vi "Drive Controller.vi"(8 "error in":errorcluster) -> ()   [LabVIEW 2015]
doc: "This VI executes continuously carrying out the current operation and responding to updates or new operation requests. It will often contain the timing or control code that is difficult to place directly in TeleOp. This VI generally opens all sensors and motors and isolates the rest of the robot code from knowing implementation details of how the operations are carried out."
uses:
  <vilib>/Rock Robotics/WPI/CAN/TalonSRX/WPI_CANTalonSRX_GlobalStatus.ctl
  Drive Setpoints.ctl
  Drive Operations.ctl
  <vilib>/Rock Robotics/WPI/CAN/TalonSRX/WPI_CANTalonSRX_APIControlMode.ctl
  <vilib>/Rock Robotics/WPI/SafetyOutput/WPI_SafetyOutputConfigMenu.ctl
  <vilib>/Rock Robotics/WPI/MotorControl/WPI_MotorControlOpenCANTalonSRX.vi
panel:
  out "Talon SRX Status":T1
  out "Setpoints":T2(graph)
  out "Current\nCmd":string
  # "Tip: It may be helpful to observe inputs and sensor values.\nYou may also want to display tuning or debugging controls."
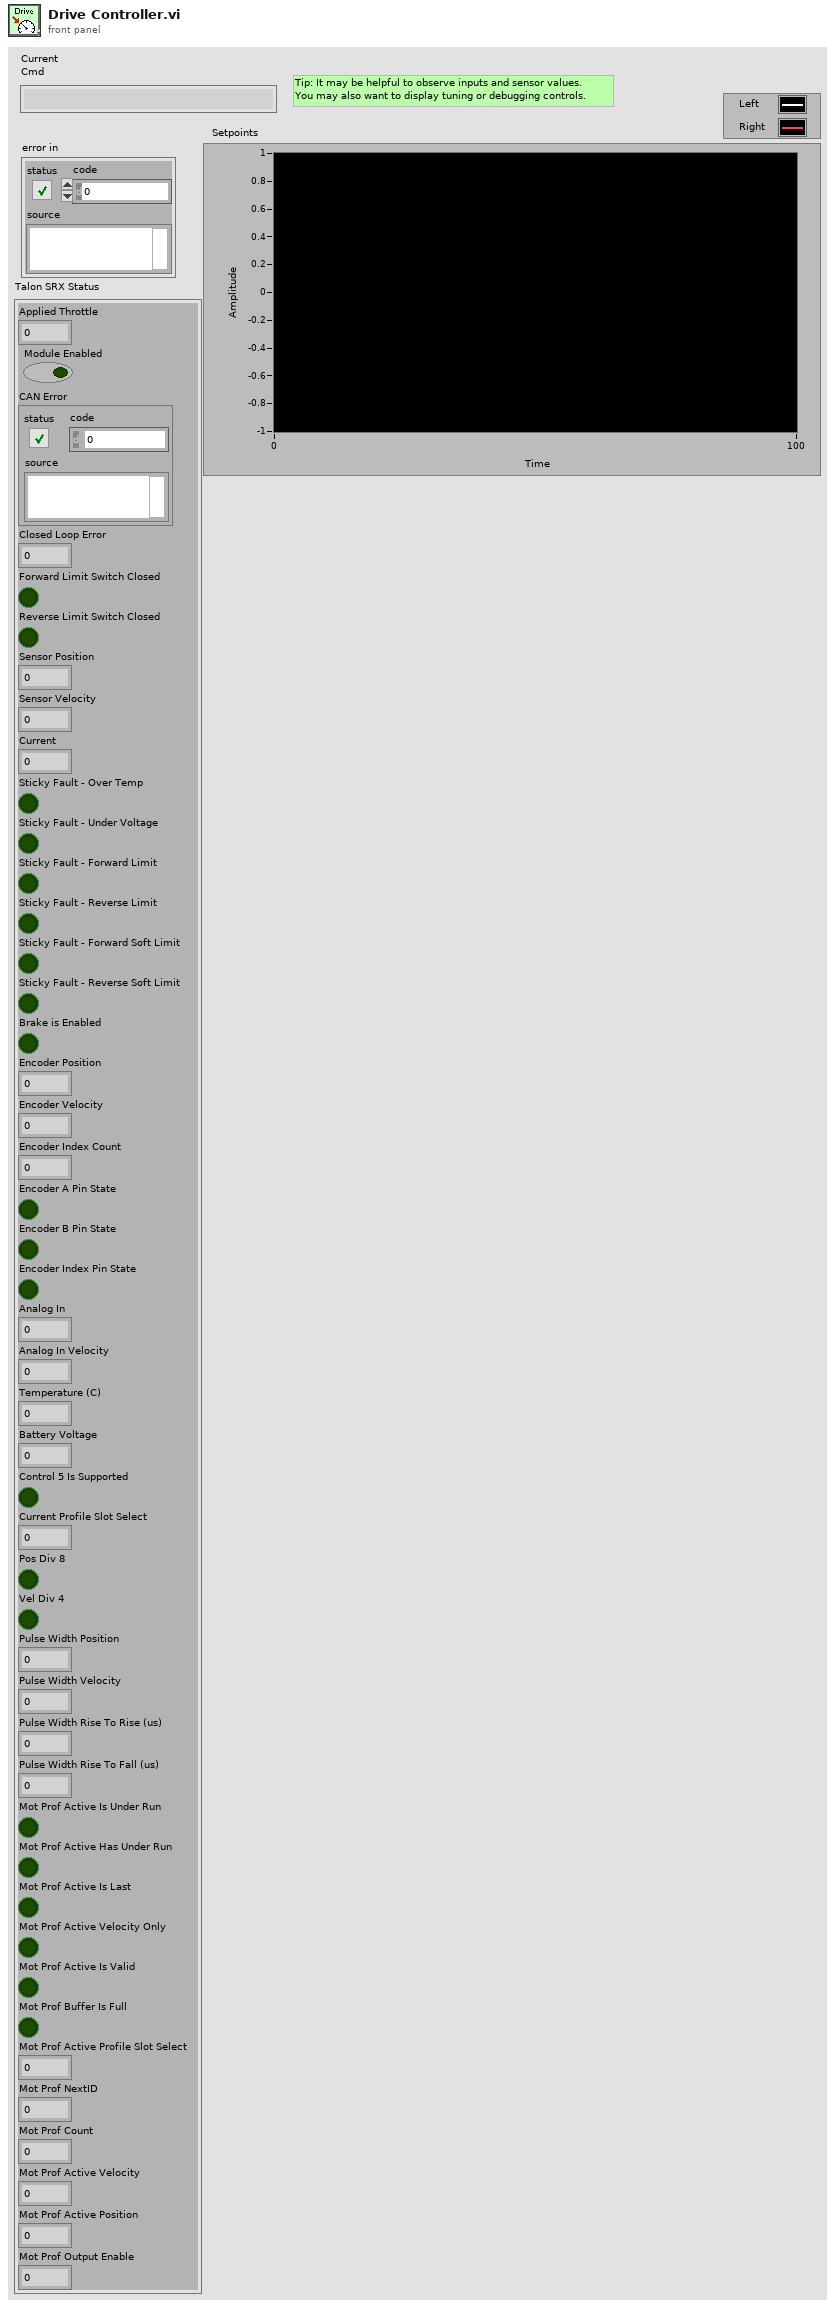
[diagram p1: front panel]
types:
  T1 = typedef "WPI_CANTalonSRX_GlobalStatus.ctl" = cluster{"Applied Throttle":dbl, "Module Enabled":bool, "CAN Error":errorcluster, "Closed Loop Error":dbl, "Forward Limit Switch Closed":bool, "Reverse Limit Switch Closed":bool, "Sensor Position":dbl, "Sensor Velocity":dbl, "Current":dbl, "Sticky Fault - Over Temp":bool, "Sticky Fault - Under Voltage":bool, "Sticky Fault - Forward Limit":bool, "Sticky Fault - Reverse Limit":bool, "Sticky Fault - Forward Soft Limit":bool, "Sticky Fault - Reverse Soft Limit":bool, "Brake is Enabled":bool, "Encoder Position":dbl, "Encoder Velocity":dbl, "Encoder Index Count":dbl, "Encoder A Pin State":bool, "Encoder B Pin State":bool, "Encoder Index Pin State":bool, "Analog In":dbl, "Analog In Velocity":dbl, "Temperature (C)":dbl, "Battery Voltage":dbl, "Control 5 Is Supported":bool, "Current Profile Slot Select":dbl, "Pos Div 8":bool, "Vel Div 4":bool, "Pulse Width Position":i32, "Pulse Width Velocity":i32, "Pulse Width Rise To Rise (us)":i32, "Pulse Width Rise To Fall (us)":i32, "Mot Prof Active Is Under Run":bool, "Mot Prof Active Has Under Run":bool, "Mot Prof Active Is Last":bool, "Mot Prof Active Velocity Only":bool, "Mot Prof Active Is Valid":bool, "Mot Prof Buffer Is Full":bool, "Mot Prof Active Profile Slot Select":i32, "Mot Prof NextID":i32, "Mot Prof Count":i32, "Mot Prof Active Velocity":dbl, "Mot Prof Active Position":dbl, "Mot Prof Output Enable":i32}
  T2 = cluster{"Left Setpoint":dbl, "Right Setpoint":dbl}
  T3 = typedef "WPI_CANTalonSRX_APIControlMode.ctl" = enum8{"Percent VBus", "Speed", "Position", "Slave", "Unchanged / Invalid", "Voltage Compensation", "Current", "Motion Profile"}
  T4 = typedef "WPI_SafetyOutputConfigMenu.ctl" = enum16{"Enable", "Disable"}
  T5 = typedef "Drive Setpoints.ctl" = cluster{"Operation":T6, "Left Setpoint":dbl, "Right Setpoint":dbl, "Duration":dbl}
  T6 = typedef "Drive Operations.ctl" = enum16{"Reserve", "Read Current", "Immediate", "Drive for Time", "Drive for Distance"}
  T7 = typedef "WPI_MotorControlDeviceRef.ctl" = cluster{"DeviceStatus":errorcluster, "Type":T8, "PWM":cluster{"PWM Channel":T9, "DeadBand":T10}, "CAN":cluster{"Device Number":u8, "Control Mode":T11, "Semaphore":T12, "Max Vout":dbl, "TalonSRX Control Mode":T3}, "Invert":bool}
  T8 = typedef "WPI_MotorControlType.ctl" = enum16{"PWM", "CAN", "CANTalonSRX"}
  T9 = typedef "FPGA_DIOPWMChannel.ctl" = enum8{"PWM 0", "PWM 1", "PWM 2", "PWM 3", "PWM 4", "PWM 5", "PWM 6", "PWM 7", "PWM 8", "PWM 9", "PWM MXP 0", "PWM MXP 1", "PWM MXP 2", "PWM MXP 3", "PWM MXP 4", "PWM MXP 5", "PWM MXP 6", "PWM MXP 7", "PWM MXP 8", "PWM MXP 9", "Invalid"}
  T10 = typedef "WPI_PWMDeadband.ctl" = cluster{"Name":string, "maxPositivePwm":i32, "minPositivePwm":i32, "centerPwm":i32, "maxNegativePwm":i32, "minNegativePwm":i32, "angularRange":u16}
  T11 = typedef "WPI_CANJaguar_ControlMode.ctl" = enum8{"Percent VBus", "Current", "Speed", "Position", "Voltage"}
  T12 = typedef "Semaphore RefNum" = refnum<k1>
  T13 = typedef "Command Status Info.ctl" = cluster{"Name":string, "Status":T14, "notifier out":T15}
  T14 = typedef "Completion Status.ctl" = enum16{"Successful", "Aborted", "Incomplete"}
  T15 = typedef "Completion Notifier.ctl" = refnum<notifier>
  T16 = cluster{"SubSystem Data":T5, cluster{"Start Time (ms)":u32, "Iterations":i32}, cluster{"Command Info":T13, "Description":string, "SubSystem Data":T5, "notifier out":refnum<notifier>, "Subsystem Name":string}}
  T17 = cluster{"SubSystem Data":T5, cluster{"Start Time (ms)":u32, "Iterations":i32}, "Default Command Arguments":cluster{"Command Info":T13, "Description":string, "SubSystem Data":T5, "notifier out":refnum<notifier>, "Subsystem Name":string}}
  T18 = cluster{"Don't move motors while reserved":dbl, "Don't move motors while reserved":dbl}
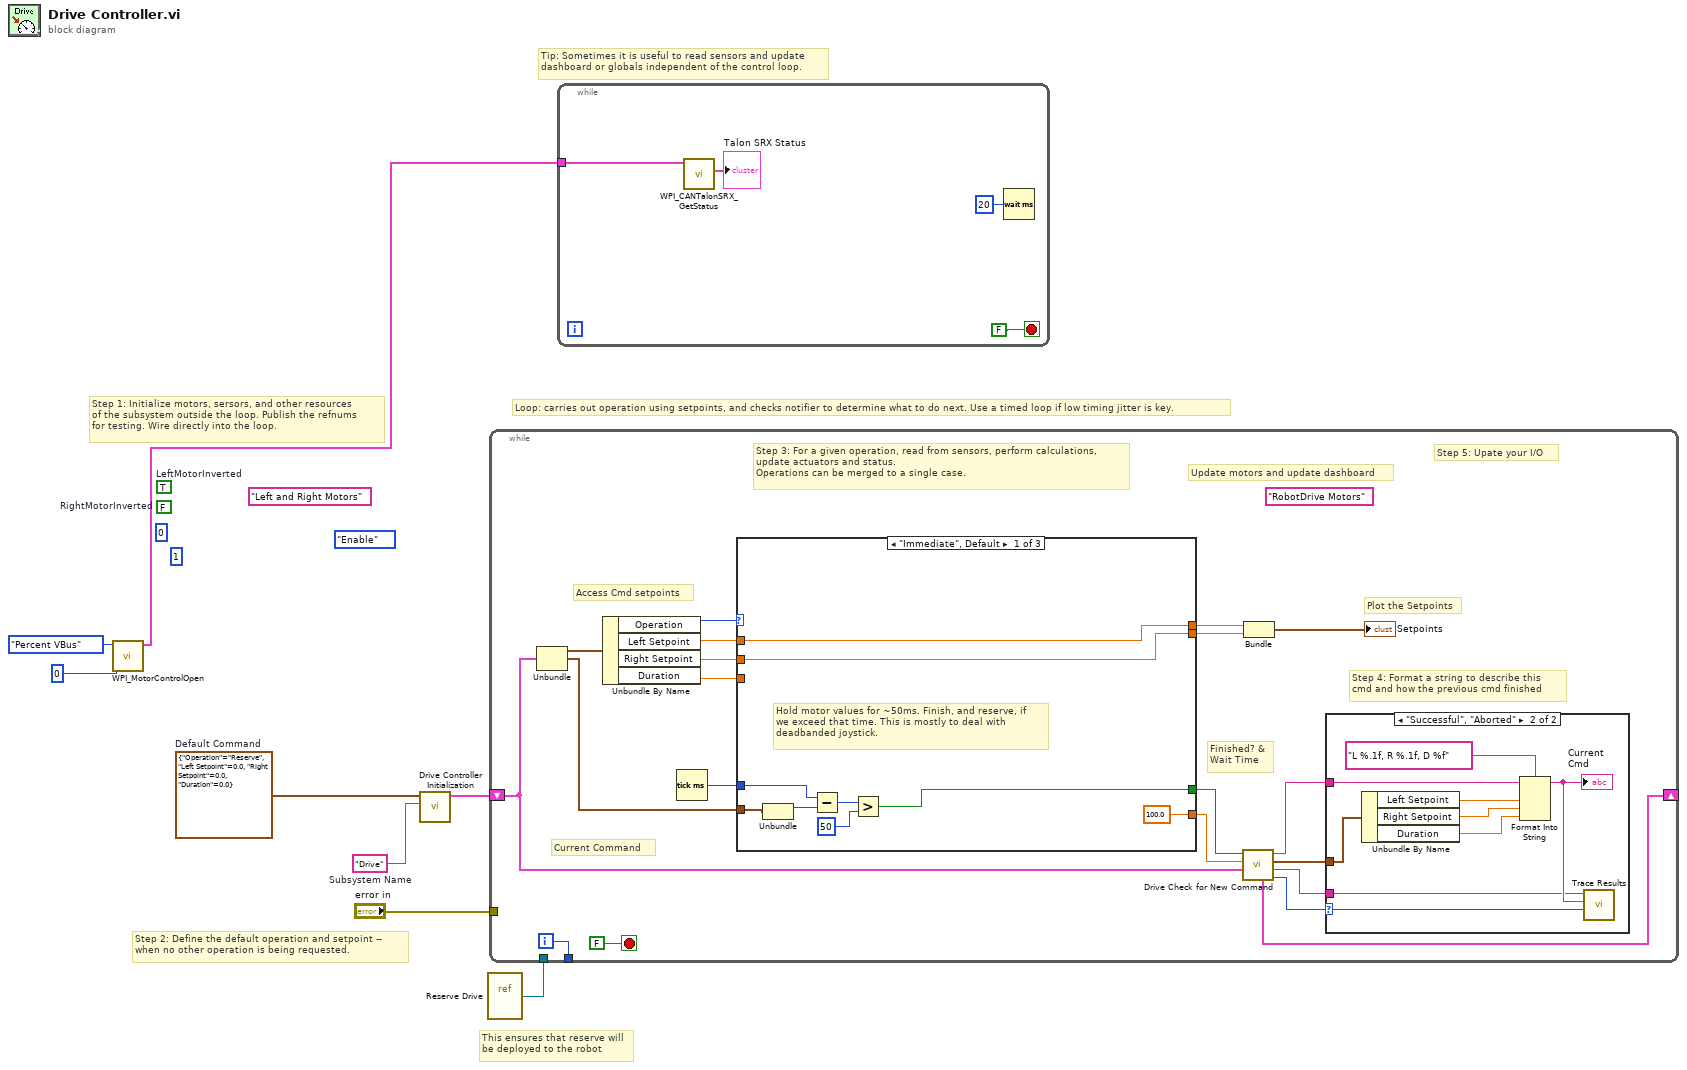
[diagram p0: block diagram]
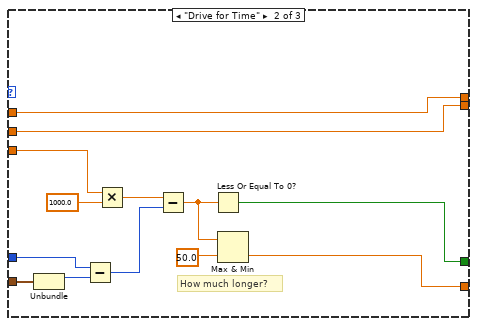
[diagram p3: hidden frame]
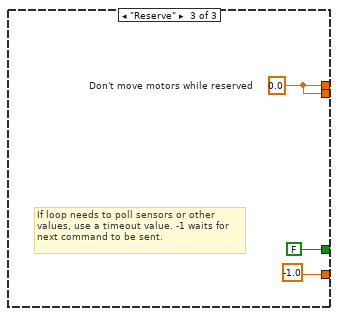
[diagram p4: hidden frame]
diagram:
  (unwired) u8 1 ("Left Motor")
  (unwired) u8 0 ("Left Motor")
  (unwired) WPI_SafetyOutputConfigMenu."Enable" ("mode")
  (unwired) "Left and Right Motors" ("refnum name")
  (unwired) TRUE  # LeftMotorInverted
  (unwired) FALSE  # RightMotorInverted
  w7 = T5 {"Operation"=enum."Reserve", "Left Setpoint"=0.0, "Right Setpoint"=0.0, "Duration"=0.0}  # Default Command
  w8 = "Drive"  # Subsystem Name
  # "This ensures that reserve will\nbe deployed to the robot"
  # "Tip: Sometimes it is useful to read sensors and update\ndashboard or globals independent of the control loop."
  # "Step 2: Define the default operation and setpoint --\nwhen no other operation is being requested."
  # "Step 1: Initialize motors, sersors, and other resources\nof the subsystem outside the loop. Publish the refnums\nfor testing. Wire directly into the loop."
  # "Loop: carries out operation using setpoints, and checks notifier to determine what to do next. Use a timed loop if low timing jitter is key."
  n1 = call-poly <vilib>:"WPI_MotorControlOpen.vi"("Device Number"=u8 0, "Control Mode"=WPI_CANTalonSRX_APIControlMode."Percent VBus") -> ("MotorControlDeviceRef"=w1:T7)  [unwired: 8 in, 1 out]
  n2 = call "Drive Controller Initialization.vi"("Subsystem Name"=w8, "Default Command"=w7) -> ("output cluster"=w5:T16)  [unwired: 9 in]
  n3 = vi-ref "Reserve Drive.vi"() -> (w4:refnum<vi>)
  n4 = while {
    shift-right: [w16] -> _
    shift-left: w5 -> [w9]
    tunnel: [w27] -> _
    tunnel: "error in" -> [_]
    tunnel: w4 -> [_]
    i -> [w27]
    stop <- FALSE stop-if-true
    (unwired) "RobotDrive Motors" ("Name")
    # "Step 5: Upate your I/O"
    # "Step 4: Format a string to describe this\ncmd and how the previous cmd finished"
    # "Current Command"
    # "Update motors and update dashboard"
    # "Plot the Setpoints"
    # "Access Cmd setpoints"
    # "Finished? &\nWait Time"
    # "Step 3: For a given operation, read from sensors, perform calculations,\nupdate actuators and status.\nOperations can be merged to a single case."
    n5 = Unbundle(w9) -> ("SubSystem Data"=w23:T5, w10:cluster{"Start Time (ms)":u32, "Iterations":i32})  [unwired: 1 out]
    n6 = Unbundle By Name(w23) -> ("Operation"=w22:T6, "Left Setpoint"=w21:dbl, "Right Setpoint"=w20:dbl, "Duration"=w19:dbl)
    n7 = Tick Count (ms)() -> (millisecond timer value=w18:u32)
    n8 = case shown="\"Immediate\", Default" w22 {
      tunnel: [100.0 w47 -1.0] -> w15
      tunnel: [w39 w54 FALSE ("ignore previous (F)")] -> w14
      tunnel: w10 -> [w38 w56 _]
      tunnel: [w45 w53 w60] -> w25
      tunnel: [w44 w52 w60] -> w24
      tunnel: w21 -> [w45 w53 _]
      tunnel: w20 -> [w44 w52 _]
      tunnel: w19 -> [_ w51 _]
      tunnel: w18 -> [w40 w50 _]
      frame "Immediate", Default {
        # "Hold motor values for ~50ms. Finish, and reserve, if\nwe exceed that time. This is mostly to deal with\ndeadbanded joystick."
        n9 = Unbundle(w38) -> ("Start Time (ms)"=w41:u32)  [unwired: 1 out]
        n10 = Subtract(x=w40, y=w41) -> (x-y=w42:u32)
        n11 = Greater?(x=w42, y=u8 50 ("Left Motor")) -> (0:w39:bool)
      }
      frame "Drive for Time" {
        # "How much longer?"
        n12 = Unbundle(w56) -> ("Start Time (ms)"=w55:u32)  [unwired: 1 out]
        n13 = Subtract(x=w50, y=w55) -> (x-y=w59:u32)
        n14 = Multiply(x=w51, y=1000.0) -> (x*y=w58:dbl)
        n15 = Subtract(x=w58, y=w59) -> (x-y=w49:dbl)
        n16 = Less Or Equal To 0?(x=w49) -> (x <= 0?=w54:bool)
        n17 = Max & Min(x=w49, y=50.0) -> (min(x,y)=w47:dbl)  [unwired: 1 out]
      }
      frame "Reserve" {
        w60 = 0.0  # Don't move motors while reserved
        # "If loop needs to poll sensors or other\nvalues, use a timeout value. -1 waits for\nnext command to be sent."
      }
    }
    n18 = call "Drive Check for New Command.vi"("input cluster"=w9, "Wait time (ms)"=w15, "Finished?"=w14) -> ("Completion"=w17:T14, "Subsystem Name"=w11:string, "SetPoint"=w12:T5, "Initial Trace String"=w13:string, "output cluster"=w16:T17)  [unwired: 4 in]
    n19 = Bundle("Don't move motors while reserved"=w25, "Don't move motors while reserved"=w24) -> (→"Setpoints":T18)  [unwired: 1 in]
    n20 = case shown="\"Successful\", \"Aborted\"" w17 {
      selector: w17 -> [_ w37]
      tunnel: w13 -> [_ w32]
      tunnel: w12 -> [_ w33]
      tunnel: w11 -> [_ w29]
      frame "Incomplete", Default {
        # "Continuing current command"
      }
      frame "Successful", "Aborted" {
        # "Report and setup for next command"
        n21 = Unbundle By Name(w33) -> ("Left Setpoint"=w35:dbl, "Right Setpoint"=w36:dbl, "Duration"=w30:dbl)
        n22 = Format Into String(format string="L %.1f, R %.1f, D %f", initial string=w32, w35, w36, w30) -> (resulting string=w31:string)  [unwired: 1 in, 1 out]
        "Current\nCmd" <- w31
        n23 = call <vilib>:"Trace Results.vi"("Status of previous command"=w37, "Description"=w31, "Subsystem"=w29) -> ()  [unwired: 9 in]
      }
    }
  }
  n24 = while {
    tunnel: w1 -> [w64]
    stop <- FALSE stop-if-true
    n25 = call <vilib>:"WPI_CANTalonSRX_GetStatus.vi"("CAN Talon SRX Ref"=w64) -> ("Talon SRX Status"=→"Talon SRX Status":T1)  [unwired: 8 in, 2 out]
    n26 = Wait (ms)(milliseconds to wait=u32 20) -> ()  [unwired: 1 out]
  }
